vi "Read Net Config.vi"(8 "error in (no error)":errorcluster, 9 "Node Config in":refnum<class "Node Config.lvclass">, 10 "Config Element in":refnum<class "Config Element.lvclass">, 11 "Node in":refnum<class "Node Config.lvclass">) -> (0 "error out":errorcluster, 1 "Node Config out":refnum<class "Node Config.lvclass">, 3 "Node out":refnum<class "Node Config.lvclass">)   [LabVIEW 2020, in "VolatusConfig.lvlib" / "Node Config.lvclass"]
uses:
  Node Config.lvclass
  lv-vecto/Vecto/Node Config/Node Config.lvclass
  lv-cdm/CDM-Config/Config Element/Config Element.lvclass
  lv-vecto/Vecto/Node Config/TCP Messaging Info.ctl
  lv-vecto/Vecto/Node Config/HTTP Server Info.ctl
  Node Config.lvclass/Node Config.ctl
  lv-vecto/VectoConfig/VectoConfig.lvlib
  lv-vecto/Vecto/IP Resolver/IP Resolver.lvclass
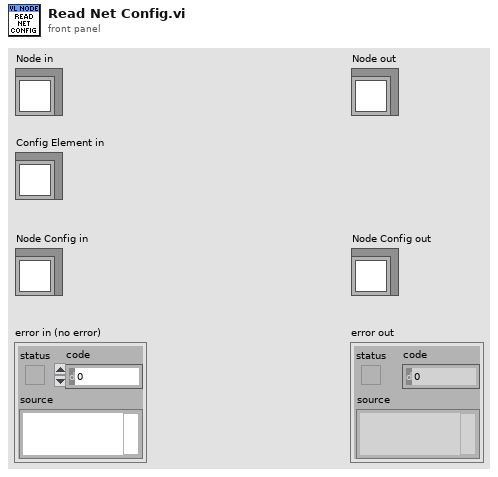
[diagram p1: front panel]
types:
  T1 = typedef "CDM-Config.lvlib/Value Type.ctl" = enum16{"String", "Number", "Bool", "Object", "Array"}
  T2 = typedef "VectoConfig.lvlib/TCP Messaging Info.ctl" = cluster{"Address":string, "Port":u16, "Server (Client)":bool}
  T3 = typedef "VectoConfig.lvlib/HTTP Server Info.ctl" = cluster{"HTTP Port":u16, "Debug":bool}
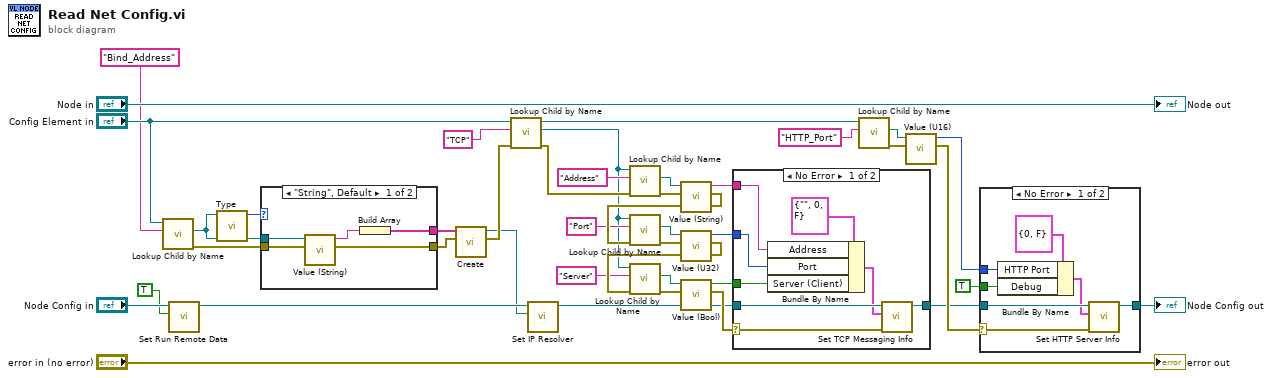
[diagram p0: block diagram]
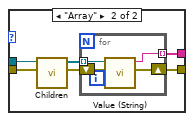
[diagram p2: hidden frame]
diagram:
  n1 = call "Lookup Child by Name.vi"("Name"="Bind_Address", "Config Element in"="Config Element in") -> ("error out"=w6:errorcluster, "Child"=w7:refnum<class "Config Element.lvclass">)  [unwired: 6 in, 2 out]
  n2 = call "Set Run Remote Data.vi"("Run Remote Data"=TRUE, "Node Config in"="Node Config in") -> ("Node Config out"=w5:refnum<class "Node Config.lvclass">)  [unwired: 8 in, 1 out]
  n3 = call "Type.vi"("Config Element in"=w7) -> ("Value Type"=w8:T1)  [unwired: 9 in, 1 out]
  n4 = case shown="\"String\", Default" w8 {
    tunnel: w7 -> [w47 w53]
    tunnel: w6 -> [w46 w51]
    tunnel: [w45 w49] -> w2
    tunnel: [w43 w48] -> w1
    frame "String", Default {
      n5 = call "Value (String).vi"("error in (no error)"=w46, "Config Element in"=w47) -> ("error out"=w43:errorcluster, "String Value"=w44:string)  [unwired: 8 in]
      n6 = Build Array(w44) -> (w45:string[])
    }
    frame "Array" {
      n7 = call "Children.vi"("error in (no error)"=w51, "Config Element in"=w53) -> ("error out"=w50:errorcluster, "Elements"=w52:refnum<class "Config Element.lvclass">[])  [unwired: 8 in]
      n8 = for {
        tunnel: w52 -> [w57] mode=indexing
        shift-right: [w55] -> w48
        shift-left: w50 -> [w56]
        tunnel: [w54] -> w49 mode=indexing
        n9 = call "Value (String).vi"("error in (no error)"=w56, "Config Element in"=w57) -> ("error out"=w55:errorcluster, "String Value"=w54:string)  [unwired: 8 in]
      }
    }
  }
  n10 = call "Create.vi"("error in (no error)"=w1, "Bindings"=w2) -> ("error out"=w42:errorcluster, "IP Resolver"=w4:refnum<class "IP Resolver.lvclass">)  [unwired: 8 in]
  n11 = call "Lookup Child by Name.vi"("error in (no error)"=w42, "Name"="TCP", "Config Element in"="Config Element in") -> ("error out"=w28:errorcluster, "Child"=w10:refnum<class "Config Element.lvclass">, "Config Element out"=w16:refnum<class "Config Element.lvclass">)  [unwired: 5 in, 1 out]
  n12 = call "Set IP Resolver.vi"("IP Resolver"=w4, "Node Config in"=w5) -> ("Node Config out"=w3:refnum<class "Node Config.lvclass">)  [unwired: 8 in, 1 out]
  n13 = call "Lookup Child by Name.vi"("error in (no error)"=w28, "Name"="Address", "Config Element in"=w10) -> ("error out"=w29:errorcluster, "Child"=w30:refnum<class "Config Element.lvclass">)  [unwired: 5 in, 2 out]
  n14 = call "Value (String).vi"("error in (no error)"=w29, "Config Element in"=w30) -> ("error out"=w27:errorcluster, "String Value"=w20:string)  [unwired: 8 in]
  n15 = call "Lookup Child by Name.vi"("error in (no error)"=w27, "Name"="Port", "Config Element in"=w10) -> ("error out"=w25:errorcluster, "Child"=w24:refnum<class "Config Element.lvclass">)  [unwired: 5 in, 2 out]
  n16 = call "Value (U32).vi"("error in (no error)"=w25, "Config Element in"=w24) -> ("error out"=w34:errorcluster, "U32 Value"=w19:u32)  [unwired: 8 in]
  n17 = call "Lookup Child by Name.vi"("error in (no error)"=w34, "Name"="Server", "Config Element in"=w10) -> ("error out"=w22:errorcluster, "Child"=w23:refnum<class "Config Element.lvclass">)  [unwired: 5 in, 2 out]
  n18 = call "Value (Bool).vi"("error in (no error)"=w22, "Config Element in"=w23) -> ("error out"=w35:errorcluster, "Bool Value"=w18:bool)  [unwired: 8 in]
  n19 = case shown="No Error" w35 {
    selector: w35 -> [w58 _]
    tunnel: w3 -> [w65 w66]
    tunnel: [w64 w66] -> w17
    tunnel: w20 -> [w61 _]
    tunnel: w19 -> [w60 _]
    tunnel: w18 -> [w59 _]
    frame No Error {
      n20 = Bundle By Name(cluster=T2 {"Address"="", "Port"=0, "Server (Client)"=FALSE} ("TCP Messaging Info"), "Address"=w61, "Port"=w60, "Server (Client)"=w59) -> (w62:T2)
      n21 = call "Set TCP Messaging Info.vi"("error in (no error)"=w58, "TCP Messaging Info"=w62, "Node Config in"=w65) -> ("Node Config out"=w64:refnum<class "Node Config.lvclass">)  [unwired: 7 in, 1 out]
    }
    frame Error {
    }
  }
  n22 = call "Lookup Child by Name.vi"("Name"="HTTP_Port", "Config Element in"=w16) -> ("error out"=w11:errorcluster, "Child"=w14:refnum<class "Config Element.lvclass">)  [unwired: 6 in, 2 out]
  n23 = call "Value (U16).vi"("error in (no error)"=w11, "Config Element in"=w14) -> ("error out"=w36:errorcluster, "U16 Value"=w12:u16)  [unwired: 8 in]
  n24 = case shown="No Error" w36 {
    selector: w36 -> [w67 _]
    tunnel: w17 -> [w73 w74]
    tunnel: TRUE ("Debug") -> [w70 _]
    tunnel: w12 -> [w69 _]
    tunnel: [w68 w74] -> w38
    frame No Error {
      n25 = Bundle By Name(cluster=T3 {"HTTP Port"=0, "Debug"=FALSE} ("HTTP Server Info"), "HTTP Port"=w69, "Debug"=w70) -> (w71:T3)
      n26 = call "Set HTTP Server Info.vi"("error in (no error)"=w67, "HTTP Server Info"=w71, "Node Config in"=w73) -> ("Node Config out"=w68:refnum<class "Node Config.lvclass">)  [unwired: 7 in, 1 out]
    }
    frame Error {
    }
  }
  "Node Config out" <- w38
  "error out" <- "error in (no error)"
  "Node out" <- "Node in"
